vi "GetOptions.vi"() -> ()   [LabVIEW 2012]
panel:
  out "Current Setting":string
  in  "Enum":T1(ring)
  out "error out":errorcluster
  out "Options":string[](array[string])
  out "index":i32
  out "SerialNumber":string
  in  "error in (no error)":errorcluster
  in  "OphirComRef":refnum<k7>
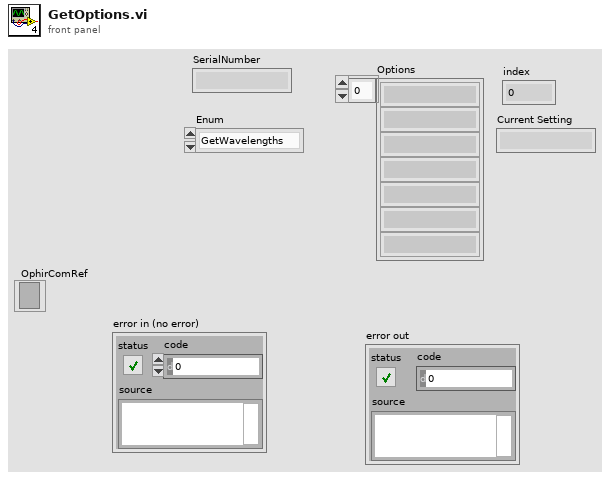
[diagram p1: front panel]
types:
  T1 = enum16{"GetWavelengths", "GetRanges", "GetMode", "GetFilter"}
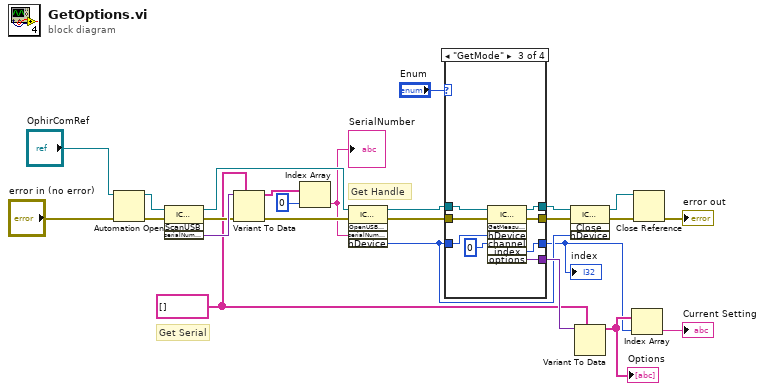
[diagram p0: block diagram]
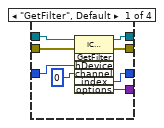
[diagram p2: hidden frame]
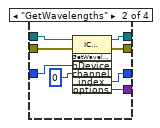
[diagram p3: hidden frame]
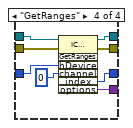
[diagram p4: hidden frame]
diagram:
  w12 = string[] []
  # "Get Handle"
  # "Get Serial"
  n1 = Automation Open(error in (no error)="error in (no error)", Automation Refnum="OphirComRef") -> (Automation Refnum=w23:refnum<k7>, error out=w19:errorcluster)  [unwired: 2 in]
  n2 = invoke class="ICoLMMeasurement" method="ScanUSB"(reference=w23, error in=w19) -> (reference out=w17:refnum<k7>, error out=w20:errorcluster, "serialNumbers"=w22:variant)  [unwired: 2 in, 1 out]
  n3 = Variant To Data(error in=w20, type=w12, Variant=w22) -> (data=w21:string[], error out=w16:errorcluster)
  n4 = Index Array(array=w21, index=0) -> (element=w15:string)
  "SerialNumber" <- w15
  n5 = invoke class="ICoLMMeasurement" method="OpenUSBDevice"(reference=w17, error in=w16, "serialNumber"=w15) -> (reference out=w14:refnum<k7>, error out=w8:errorcluster, "hDevice"=w11:i32)  [unwired: 2 in, 2 out]
  n6 = case shown="\"GetMode\"" "Enum" {
    tunnel: w14 -> [w33 w41 w42 w57]
    tunnel: [w31 w37 w47 w55] -> w2
    tunnel: [w32 w38 w48 w54] -> w13
    tunnel: w11 -> [w30 w40 w46 w53]
    tunnel: [w28 w34 w49 w52] -> w10
    tunnel: [w27 w36 w43 w51] -> w9
    tunnel: w8 -> [w26 w35 w44 w50]
    frame "GetFilter", Default {
      n7 = invoke class="ICoLMMeasurement" method="GetFilter"(reference=w33, error in=w26, "hDevice"=w30, "channel"=0) -> (reference out=w28:refnum<k7>, error out=w27:errorcluster, "index"=w31:i32, "options"=w32:variant)  [unwired: 3 in, 3 out]
    }
    frame "GetWavelengths" {
      n8 = invoke class="ICoLMMeasurement" method="GetWavelengths"(reference=w41, error in=w35, "hDevice"=w40, "channel"=0) -> (reference out=w34:refnum<k7>, error out=w36:errorcluster, "index"=w37:i32, "options"=w38:variant)  [unwired: 3 in, 3 out]
    }
    frame "GetMode" {
      n9 = invoke class="ICoLMMeasurement" method="GetMeasurementMode"(reference=w42, error in=w44, "hDevice"=w46, "channel"=0) -> (reference out=w49:refnum<k7>, error out=w43:errorcluster, "index"=w47:i32, "options"=w48:variant)  [unwired: 3 in, 3 out]
    }
    frame "GetRanges" {
      n10 = invoke class="ICoLMMeasurement" method="GetRanges"(reference=w57, error in=w50, "hDevice"=w53, "channel"=0) -> (reference out=w52:refnum<k7>, error out=w51:errorcluster, "index"=w55:i32, "options"=w54:variant)  [unwired: 3 in, 3 out]
    }
  }
  "index" <- w2
  n11 = invoke class="ICoLMMeasurement" method="Close"(reference=w10, error in=w9, "hDevice"=w11) -> (reference out=w7:refnum<k7>, error out=w6:errorcluster)  [unwired: 1 in, 2 out]
  n12 = Variant To Data(type=w12, Variant=w13) -> (data=w3:string[])  [unwired: 1 in, 1 out]
  "Options" <- w3
  n13 = Index Array(array=w3, index=w2) -> (element=→"Current Setting":string)
  n14 = Close Reference(reference=w7, error in (no error)=w6) -> (error out=→"error out":errorcluster)
